vi "Run Fix Operation.vi"(8 "error in":errorcluster, 10 "Run Chamber":bool=TRUE, 11 "VISA resource name":refnum<visa-resource-name>) -> (0 "error out":errorcluster, 2 "Successfully":bool, 3 "VISA resource name out":refnum<visa-resource-name>)   [LabVIEW 2017, in "Samwontech TEMP2xxx.lvlib"]
doc: "Activate FIX operation Run"
uses:
  <instrlib>/Samwontech TEMP2xxx/Samwontech TEMP2xxx.lvlib
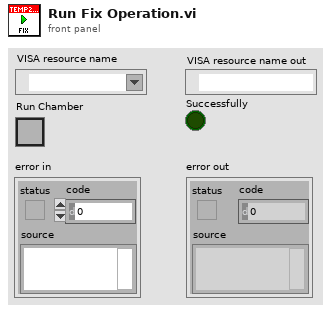
[diagram p1: front panel]
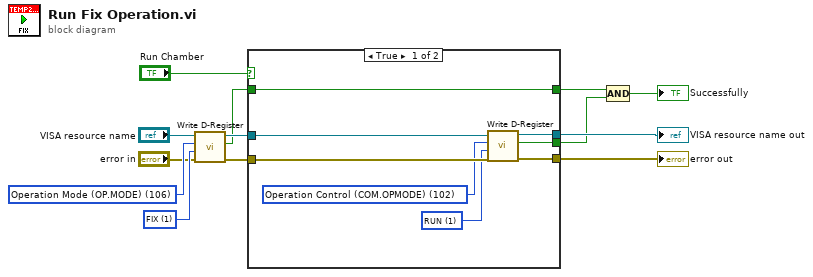
[diagram p0: block diagram]
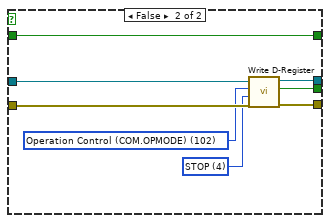
[diagram p2: hidden frame]
diagram:
  w11 = u32 1 items=["PROG", "FIX"] ("Operation Mode")
  w12 = u32 106 items=["Current PV (NPV)"=1, "Operation Control (COM.OPMODE)"=102, "Set Point on FIX operation (FIX.TSP)"=104, "Operation Mode (OP.MODE)"=106] ("D-Registers Map")
  n1 = call <instrlib>:"Write D-Register.vi"("error in"="error in", "Data"=w11, "D-register number"=w12, "VISA resource name"="VISA resource name") -> ("error out"=w9:errorcluster, "Successfully"=w3:bool, "VISA resource name out"=w10:refnum<visa-resource-name>)  [unwired: 4 in, 1 out]
  n2 = case shown="True" "Run Chamber" {
    tunnel: w10 -> [w21 w29]
    tunnel: w9 -> [w20 w28]
    tunnel: [w17 w25] -> w4
    tunnel: [w16 w24] -> w5
    tunnel: [w15 w23] -> w1
    tunnel: w3 -> [w14 w22]
    tunnel: [w14 w22] -> w2
    frame True {
      w18 = u32 1 items=["RUN"=1, "HOLD"=2, "STEP"=3, "STOP"=4] ("Mode Control")
      w19 = u32 102 items=["Current PV (NPV)"=1, "Operation Control (COM.OPMODE)"=102, "Set Point on FIX operation (FIX.TSP)"=104, "Operation Mode (OP.MODE)"=106] ("D-Registers Map")
      n3 = call <instrlib>:"Write D-Register.vi"("error in"=w20, "Data"=w18, "D-register number"=w19, "VISA resource name"=w21) -> ("error out"=w17:errorcluster, "Successfully"=w15:bool, "VISA resource name out"=w16:refnum<visa-resource-name>)  [unwired: 4 in, 1 out]
    }
    frame False {
      w26 = u32 4 items=["RUN"=1, "HOLD"=2, "STEP"=3, "STOP"=4] ("Mode Control")
      w27 = u32 102 items=["Current PV (NPV)"=1, "Operation Control (COM.OPMODE)"=102, "Set Point on FIX operation (FIX.TSP)"=104, "Operation Mode (OP.MODE)"=106] ("D-Registers Map")
      n4 = call <instrlib>:"Write D-Register.vi"("error in"=w28, "Data"=w26, "D-register number"=w27, "VISA resource name"=w29) -> ("error out"=w25:errorcluster, "Successfully"=w23:bool, "VISA resource name out"=w24:refnum<visa-resource-name>)  [unwired: 4 in, 1 out]
    }
  }
  "VISA resource name out" <- w5
  "error out" <- w4
  n5 = Compound Arithmetic op=AND(w2, w1) -> (→"Successfully":bool)
